vi "Single Shot Pulse Sequence.vi"() -> ()   [LabVIEW 2020]
uses:
  <instrlib>/niFgen/niFgen.llb/niFgen Waveform Type.ctl
  <instrlib>/niFgen/niFgen.llb/niFgen_ctl Trigger DigEdge - Edge Values (Ring).ctl
  <instrlib>/niFgen/niFgen.llb/niFgen_ctl Trigger Source Values (Ring).ctl
  <instrlib>/niFgen/niFgen.llb/niFgen Trigger Mode.ctl
  <instrlib>/niScope/Controls/niScope acquisition type.ctl
  <instrlib>/niScope/Controls/niScope trigger slope.ctl
  <instrlib>/niScope/Controls/niScope trigger source.ctl
  <instrlib>/niFgen/niFgen.llb/niFgen Output Mode.ctl
  <instrlib>/niScope/Configure/Trigger/niScope Configure Trigger Edge.vi
  <vilib>/Utility/file.llb/Read Delimited Spreadsheet (DBL).vi
  <instrlib>/niFgen/niFgen.llb/niFgen Create Waveform (DBL).vi
  <instrlib>/niFgen/niFgen.llb/niFgen Configure Digital Edge Start Trigger.vi
  <instrlib>/niScope/Acquire/Fetch/niScope Fetch Cluster.vi
panel:
  in  "Larmor Frequency":dbl=27465000.0 caption="Frequency" format="%.4p"
  in  "Pulse Train File":path=path "D:/Single 90 & 180 Degree Pulse Echo.txt"
  out "Pulse Echo":waveform(dbl)(graph)={"t0"=timestamp(0 s since 1904-01-01), "dt"=3.3333333333333333e-06, "Y"=array[1500 elements]} caption="Waveform Graph"
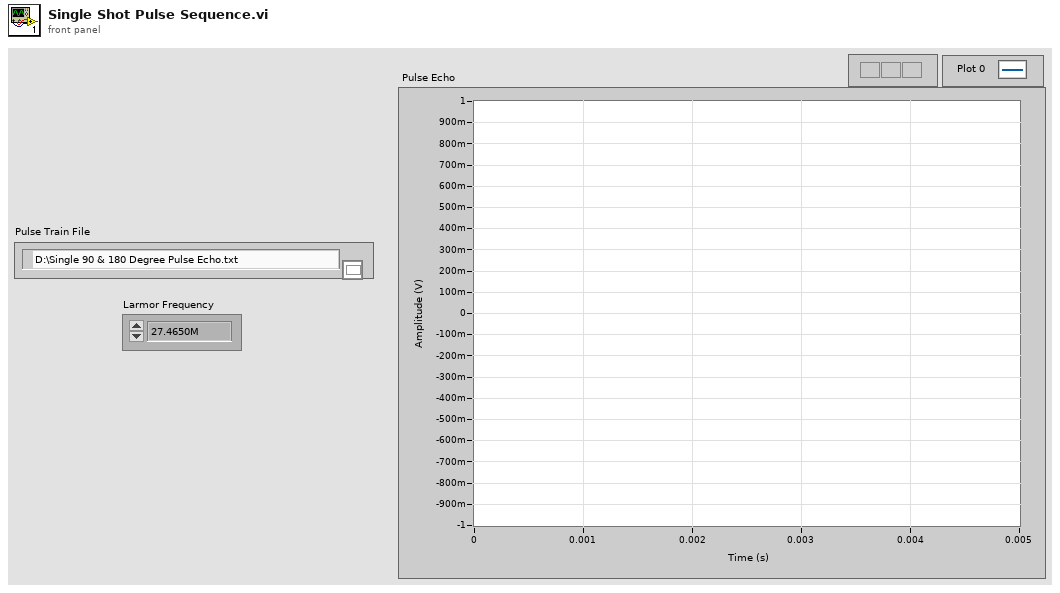
[diagram p1: front panel]
types:
  T1 = typedef "niFgen Output Mode.ctl" = u32
  T2 = typedef "niScope trigger source.ctl" = string
  T3 = typedef "niScope trigger slope.ctl" = i32
  T4 = typedef "niScope acquisition type.ctl" = i32
  T5 = typedef "niFgen Trigger Mode.ctl" = i32
  T6 = typedef "niFgen_ctl Trigger Source Values (Ring).ctl" = string
  T7 = typedef "niFgen_ctl Trigger DigEdge - Edge Values (Ring).ctl" = i32
  T8 = typedef "niFgen Waveform Type.ctl" = i32
  T9 = cluster{"relativeInitialX":dbl, "xIncrement":dbl, "wfm":dbl[]}
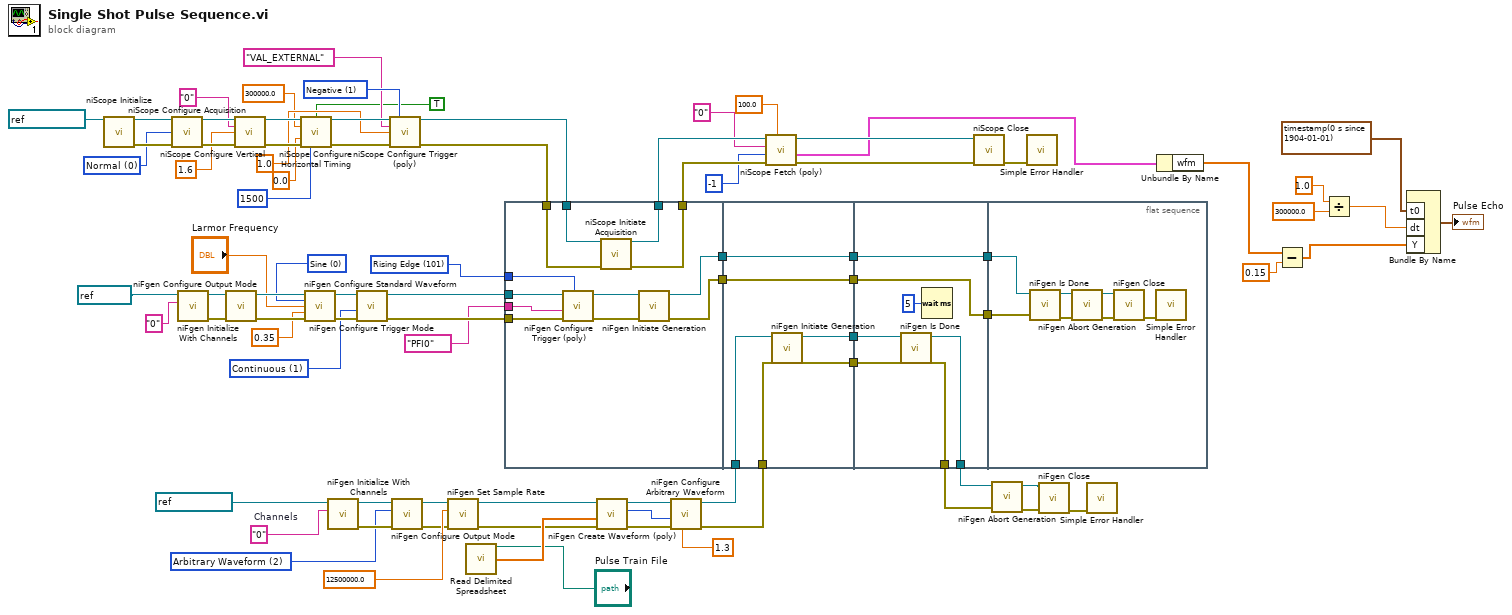
[diagram p0: block diagram]
diagram:
  w9 = "0"  # Channels
  w8 = T1 2 items=["Standard Function", "Frequency List", "Arbitrary Waveform", "Arbitrary Sequence", "Script"] ("output mode")
  w51 = T3 1 items=["Positive", "Negative"] ("trigger slope")
  w52 = T4 0 items=["Normal"=0, "Flex Res"=1, "DDC"=3] ("acquisition Type")
  w64 = T5 1 items=["Single", "Continuous", "Stepped", "Burst"] ("Trigger Mode (default: 1=continuous)")
  w68 = T7 101 items=["Rising Edge"=101, "Falling Edge"=102] ("Edge (Rising)")
  w69 = T8 0 items=["Sine", "Square", "Triangle", "Ramp Up", "Ramp Down", "DC", "Noise", "User"] ("Waveform")
  n1 = call <instrlib>:"niScope Initialize.vi"("resource name"=refnum<k15> "PXI1Slot6") -> ("instrument handle"=w53:refnum<k15>, "error out"=w54:errorcluster)  [unwired: 13 in]
  n2 = call <instrlib>:"niScope Configure Acquisition.vi"("instrument handle"=w53, "acquisition Type"=w52, "error in"=w54) -> ("instrument handle out"=w55:refnum<k15>, "error out"=w56:errorcluster)  [unwired: 11 in]
  n3 = call <instrlib>:"niFgen Initialize With Channels.vi"("Channel Name"="0", "Resource Name"=refnum<k15> "Dev1" ("Sine Wave Module")) -> ("error out"=w74:errorcluster, "Instrument Handle Out"=w77:refnum<k15>)  [unwired: 8 in]
  n4 = call <instrlib>:"niFgen Configure Output Mode.vi"("error in (no error)"=w74, "Instrument Handle"=w77) -> ("error out"=w73:errorcluster, "Instrument Handle Out"=w76:refnum<k15>)  [unwired: 7 in]
  n5 = call <instrlib>:"niScope Configure Vertical.vi"("instrument handle"=w55, "channels"="0", "vertical range"=1.6, "error in"=w56) -> ("instrument handle out"=w57:refnum<k15>, "error out"=w58:errorcluster)  [unwired: 10 in]
  n6 = call <instrlib>:"niScope Configure Horizontal Timing.vi"("instrument handle"=w57, "enforce realtime"=TRUE, "min sample rate"=300000.0, "reference position"=0.0, "error in"=w58, "min record length"=1500) -> ("instrument handle out"=w59:refnum<k15>, "error out"=w60:errorcluster)  [unwired: 8 in]
  n7 = call <instrlib>:"niFgen Configure Standard Waveform.vi"("Instrument Handle"=w76, "Waveform"=w69, "Frequency"="Larmor Frequency", "Amplitude"=0.35, "error in (no error)"=w73) -> ("Instrument Handle Out"=w75:refnum<k15>, "error out"=w72:errorcluster)  [unwired: 9 in]
  n8 = call <instrlib>:"niFgen Initialize With Channels.vi"("Channel Name"=w9, "Resource Name"=refnum<k15> "PXI1Slot3" ("FGEN Resource Name 2")) -> ("error out"=w12:errorcluster, "Instrument Handle Out"=w13:refnum<k15>)  [unwired: 8 in]
  n9 = call <instrlib>:"niFgen Configure Trigger Mode.vi"("error in (no error)"=w72, "Trigger Mode (default: 1=continuous)"=w64, "Instrument Handle"=w75) -> ("error out"=w67:errorcluster, "Instrument Handle Out"=w65:refnum<k15>)  [unwired: 7 in]
  n10 = call-poly <instrlib>:"niScope Configure Trigger (poly).vi"("instrument handle"=w59, "trigger slope"=w51, "trigger source"=T2 "VAL_EXTERNAL", "trigger level"=1.0, "error in"=w60) -> ("instrument handle out"=w45:refnum<k15>, "error out"=w44:errorcluster)  [unwired: 9 in]
  n11 = call <instrlib>:"niFgen Configure Output Mode.vi"("error in (no error)"=w12, "Output Mode (default: 0=Standard Function)"=w8, "Instrument Handle"=w13) -> ("error out"=w16:errorcluster, "Instrument Handle Out"=w15:refnum<k15>)  [unwired: 6 in]
  n12 = call <instrlib>:"niFgen Set Sample Rate.vi"("error in (no error)"=w16, "Sample Rate (Samp/s)"=12500000.0 ("Sample Rate"), "Instrument Handle"=w15) -> ("error out"=w19:errorcluster, "Instrument Handle Out"=w18:refnum<k15>)  [unwired: 7 in]
  n13 = call-poly <vilib>:"Read Delimited Spreadsheet.vi"("file path (dialog if empty)"="Pulse Train File") -> ("first row"=w20:dbl[])  [unwired: 9 in, 5 out]
  n14 = flat-sequence {
    tunnel: w68 -> [w96]
    tunnel: w67 -> [w95]
    tunnel: T6 "PFI0" ("Source") -> [w94]
    tunnel: w65 -> [w93]
    tunnel: w45 -> [w91]
    tunnel: w44 -> [w90]
    tunnel: [w89] -> w43
    tunnel: [w88] -> w42
    tunnel: [w87] -> w85
    tunnel: [w86] -> w84
    tunnel: w7 -> [w103]
    tunnel: w6 -> [w102]
    tunnel: [w101] -> w83
    tunnel: [w100] -> w82
    tunnel: [w99] -> w81
    tunnel: w85 -> [w99]
    tunnel: [w98] -> w80
    tunnel: w84 -> [w98]
    tunnel: [w109] -> w63
    tunnel: [w108] -> w62
    tunnel: w83 -> [w107]
    tunnel: w82 -> [w106]
    tunnel: [w105] -> w79
    tunnel: w81 -> [w105]
    tunnel: [w104] -> w78
    tunnel: w80 -> [w104]
    tunnel: w79 -> [w112]
    tunnel: w78 -> [w111]
    frame #0 {
      n15 = call-poly <instrlib>:"niFgen Configure Trigger (poly).vi"("Edge (Rising)"=w96, "error in (no error)"=w95, "Source"=w94, "Instrument Handle"=w93) -> ("error out"=w92:errorcluster, "Instrument Handle Out"=w97:refnum<k15>)  [unwired: 6 in]
      n16 = call <instrlib>:"niScope Initiate Acquisition.vi"("instrument handle"=w91, "error in"=w90) -> ("instrument handle out"=w89:refnum<k15>, "error out"=w88:errorcluster)  [unwired: 12 in]
      n17 = call <instrlib>:"niFgen Initiate Generation.vi"("error in (no error)"=w92, "Instrument Handle"=w97) -> ("error out"=w86:errorcluster, "Instrument Handle Out"=w87:refnum<k15>)  [unwired: 8 in]
    }
    frame #1 {
      n18 = call <instrlib>:"niFgen Initiate Generation.vi"("error in (no error)"=w103, "Instrument Handle"=w102) -> ("error out"=w100:errorcluster, "Instrument Handle Out"=w101:refnum<k15>)  [unwired: 8 in]
    }
    frame #2 {
      n19 = call <instrlib>:"niFgen Is Done.vi"("error in (no error)"=w106, "Instrument Handle"=w107) -> ("error out"=w109:errorcluster, "Instrument Handle Out"=w108:refnum<k15>)  [unwired: 7 in, 1 out]
      n20 = Wait (ms)(milliseconds to wait=u32 5) -> ()  [unwired: 1 out]
    }
    frame #3 {
      n21 = call <instrlib>:"niFgen Is Done.vi"("error in (no error)"=w111, "Instrument Handle"=w112) -> ("error out"=w115:errorcluster, "Instrument Handle Out"=w114:refnum<k15>)  [unwired: 7 in, 1 out]
      n22 = call <instrlib>:"niFgen Abort Generation.vi"("error in (no error)"=w115, "Instrument Handle"=w114) -> ("error out"=w116:errorcluster, "Instrument Handle Out"=w117:refnum<k15>)  [unwired: 8 in]
      n23 = call <instrlib>:"niFgen Close.vi"("error in (no error)"=w116, "Instrument Handle"=w117) -> ("error out"=w113:errorcluster)  [unwired: 9 in]
      n24 = call <vilib>:"Simple Error Handler.vi"("error in (no error)"=w113) -> ()  [unwired: 4 in, 5 out]
    }
  }
  n25 = call-poly <instrlib>:"niFgen Create Waveform (poly).vi"("error in (no error)"=w19, "Waveform Data Array"=w20, "Instrument Handle"=w18) -> ("error out"=w22:errorcluster, "Waveform Handle"=w23:i32, "Instrument Handle Out"=w21:refnum<k15>)  [unwired: 6 in]
  n26 = call <instrlib>:"niFgen Configure Arbitrary Waveform.vi"("Gain"=1.3, "error in (no error)"=w22, "Waveform Handle"=w23, "Instrument Handle"=w21) -> ("error out"=w7:errorcluster, "Instrument Handle Out"=w6:refnum<k15>)  [unwired: 6 in]
  n27 = call-poly <instrlib>:"niScope Fetch (poly).vi"("timeout"=100.0, "error in"=w42, "numSamples"=-1, "channels"="0", "instrument handle"=w43) -> ("error out"=w34:errorcluster, "waveform"=w32:T9, "instrument handle out"=w35:refnum<k15>)  [unwired: 3 in, 1 out]
  n28 = call <instrlib>:"niScope Close.vi"("instrument handle"=w35, "error in"=w34) -> ("error out"=w61:errorcluster)  [unwired: 13 in]
  n29 = call <instrlib>:"niFgen Abort Generation.vi"("error in (no error)"=w63, "Instrument Handle"=w62) -> ("error out"=w1:errorcluster, "Instrument Handle Out"=w2:refnum<k15>)  [unwired: 8 in]
  n30 = call <vilib>:"Simple Error Handler.vi"("error in (no error)"=w61) -> ()  [unwired: 4 in, 5 out]
  n31 = call <instrlib>:"niFgen Close.vi"("error in (no error)"=w1, "Instrument Handle"=w2) -> ("error out"=w3:errorcluster)  [unwired: 9 in]
  n32 = call <vilib>:"Simple Error Handler.vi"("error in (no error)"=w3) -> ()  [unwired: 4 in, 5 out]
  n33 = Unbundle By Name(w32) -> ("wfm"=w25:dbl[])
  n34 = Subtract(x=w25, y=0.15) -> (x-y=w26:dbl[])
  n35 = Divide(x=1.0, y=300000.0) -> (x/y=w31:dbl)
  n36 = Bundle By Name("t0"=timestamp(0 s since 1904-01-01), "dt"=w31, "Y"=w26) -> (→"Pulse Echo":waveform(dbl))  [unwired: 1 in]
